vi "GetSensorInfo.vi"(11 "Sensor Serials IN":string[](array[string])) -> (0 "OK":bool, 1 "Sensor Types":string[](array[string]), 2 "Sensor DB IDs":string[](array[string]), 3 "Sensor Serials OUT":string[](array[string]), 4 "No. of Sensors":i32)   [LabVIEW 2019]
uses:
  <vilib>/Utility/file.llb/Read Delimited Spreadsheet (string).vi
panel:
  out "No Error?":bool=TRUE
  out "Numeric":i32
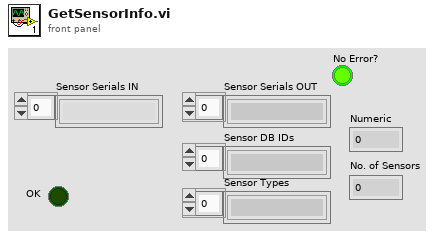
[diagram p1: front panel]
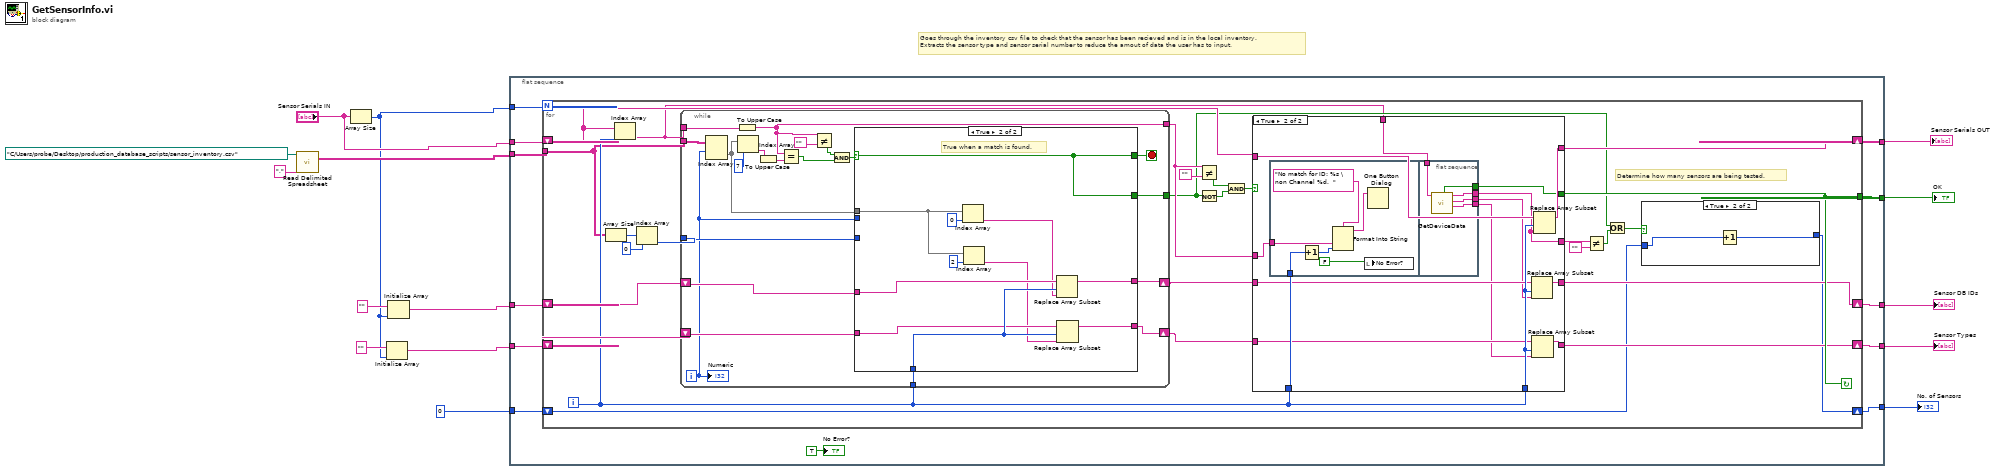
[diagram p0: block diagram]
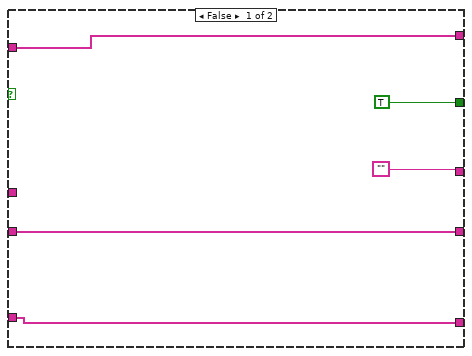
[diagram p3: hidden frame]
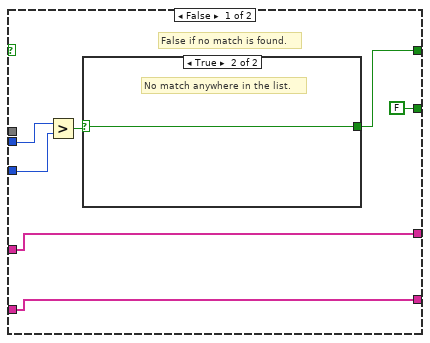
[diagram p4: hidden frame]
diagram:
  # "Goes through the inventory csv file to check that the sensor has been recieved and is in the local inventory.\nExtracts the sensor type and sensor serial number to reduce the amout of data the user has to input."
  n1 = call-poly <vilib>:"Read Delimited Spreadsheet.vi"("file path (dialog if empty)"=path "C:/Users/probe/Desktop/production_database_scripts/sensor_inventory.csv", "delimiter (\\t)"="," ("delimiter (\\t)")) -> ("all rows"=w12:string[][])  [unwired: 8 in, 5 out]
  n2 = Array Size(array="Sensor Serials IN") -> (size(s)=w9:i32)
  n3 = Initialize Array("", w9) -> (w7:string[])
  n4 = Initialize Array("", w9) -> (w8:string[])
  n5 = flat-sequence {
    tunnel: "Sensor Serials IN" -> [w27]
    tunnel: w12 -> [w26]
    tunnel: w9 -> [w25]
    tunnel: w8 -> [w24]
    tunnel: w7 -> [w23]
    tunnel: 0 -> [w17]
    tunnel: [w22] -> w6
    tunnel: [w21] -> w5
    tunnel: [w20] -> w4
    tunnel: [w19] -> w3
    tunnel: [w16] -> w1
    frame #0 {
      n6 = for {
        N: w25 -> [_]
        tunnel: w26 -> [w41]
        shift-right: [w37] -> w22
        shift-left: w24 -> [w54]
        shift-right: [w36] -> w21
        shift-left: w23 -> [w53]
        shift-right: [w47] -> w20
        shift-left: w27 -> [w48]
        tunnel: [w43] -> w19
        shift-right: [w33] -> w16
        shift-left: w17 -> [w32]
        i -> [w42]
        stop <- w43 continue-if-true
        # "Determine how many sensors are being tested."
        n7 = Array Size(array=w41) -> (size(s)=w46:i32[])
        n8 = Index Array(array=w48, index=w42) -> (element=w28:string)
        n9 = Index Array(array=w46, index=0) -> (element=w44:i32)
        n10 = while {
          tunnel: w28 -> [w107]
          tunnel: w42 -> [w103]
          tunnel: [w88] -> w40
          tunnel: [w101] -> w29
          tunnel: w44 -> [w100]
          shift-right: [w99] -> w39
          shift-left: w54 -> [w106]
          shift-right: [w102] -> w38
          shift-left: w53 -> [w105]
          tunnel: w41 -> [w97]
          i -> [w96]
          stop <- w104 stop-if-true
          n11 = Index Array(array=w97, index (row)=w96) -> (element=w95:string[])  [unwired: 1 in]
          n12 = To Upper Case(1:w107) -> (0:w88:string)
          n13 = Index Array(array=w95, index=7) -> (element=w93:string)
          n14 = To Upper Case(1:w93) -> (0:w98:string)
          n15 = Equal?(x=w88, y=w98) -> (x = y?=w90:bool)
          n16 = Not Equal?(x=w88, y="") -> (x != y?=w89:bool)
          n17 = And(x=w89, y=w90) -> (x .and. y?=w91:bool)
          n18 = case shown="True" w91 {
            selector: w91 -> [_ w117]
            tunnel: w106 -> [w114 w126]
            tunnel: w105 -> [w113 w125]
            tunnel: [w109 w117] -> w104
            tunnel: w103 -> [_ w127]
            tunnel: w95 -> [_ w124]
            tunnel: [w114 w120] -> w99
            tunnel: [w113 w119] -> w102
            tunnel: [FALSE w117] -> w101
            tunnel: w96 -> [w111 _]
            tunnel: w100 -> [w110 _]
            frame False {
              # "False if no match is found."
              n19 = Greater?(x=w111, y=w110) -> (0:w112:bool)
              n20 = case shown="True" w112 {
                selector: w112 -> [w115 w116]
                tunnel: [w115 w116] -> w109
                frame False {
                }
                frame True {
                  # "No match anywhere in the list."
                }
              }
            }
            frame True {
              # "True when a match is found."
              n21 = Index Array(array=w124, index=0) -> (element=w118:string)
              n22 = Index Array(array=w124, index=2) -> (element=w121:string)
              n23 = Replace Array Subset(array=w126, new element=w118, index=w127) -> (w120:string[])
              n24 = Replace Array Subset(array=w125, new element=w121, index=w127) -> (w119:string[])
            }
          }
          "Numeric" <- w96
        }
        n25 = Not Equal?(x=w40, y="") -> (x != y?=w50:bool)
        n26 = Not(x=w29) -> (.not. x?=w49:bool)
        n27 = And(x=w50, y=w49) -> (x .and. y?=w52:bool)
        n28 = case shown="True" w52 {
          tunnel: w42 -> [_ w73]
          tunnel: w48 -> [w62 w76]
          tunnel: [w62 w75] -> w47
          tunnel: [TRUE ("OK") w64] -> w43
          tunnel: w42 -> [_ w74]
          tunnel: w40 -> [_ w68]
          tunnel: w39 -> [w60 w72]
          tunnel: w38 -> [w59 w71]
          tunnel: [w60 w70] -> w37
          tunnel: [w59 w69] -> w36
          tunnel: ["" w65] -> w34
          tunnel: w28 -> [_ w63]
          frame False {
          }
          frame True {
            n29 = flat-sequence {
              tunnel: w74 -> [w79]
              tunnel: w68 -> [w77]
              tunnel: [w87] -> w67
              tunnel: [w86] -> w66
              tunnel: [w85] -> w65
              tunnel: [w84] -> w64
              tunnel: w63 -> [w83]
              frame #0 {
                n30 = Increment(x=w79) -> (x+1=w78:i32)
                n31 = Format Into String(format string="No match for ID: %s \non Channel %d.  " ("initial string"), w77, w78) -> (resulting string=w80:string)  [unwired: 2 in, 1 out]
                n32 = local write "No Error?"(FALSE ("Done?")) -> ()
                n33 = One Button Dialog(message=w80) -> ()  [unwired: 1 in, 1 out]
              }
              frame #1 {
                n34 = call "GetDeviceData.vi"("ID"=w83) -> ("Type 2"=w87:string, "DB Serial Number 2"=w86:string, "ID 2"=w85:string, 5:w84:bool)  [unwired: 7 in]
              }
            }
            n35 = Replace Array Subset(array=w72, new element=w66, index=w73) -> (w70:string[])
            n36 = Replace Array Subset(array=w71, new element=w67, index=w73) -> (w69:string[])
            n37 = Replace Array Subset(array=w76, new element=w65, index=w73) -> (w75:string[])
          }
        }
        n38 = Not Equal?(x=w34, y="") -> (x != y?=w30:bool)
        n39 = Or(x=w29, y=w30) -> (x .or. y?=w31:bool)
        n40 = case shown="True" w31 {
          tunnel: [w55 w57] -> w33
          tunnel: w32 -> [w55 w56]
          frame False {
          }
          frame True {
            n41 = Increment(x=w56) -> (x+1=w57:i32)
          }
        }
      }
      "No Error?" <- TRUE ("Done?")
    }
  }
  "Sensor Serials OUT" <- w4
  "Sensor DB IDs" <- w6
  "Sensor Types" <- w5
  "OK" <- w3
  "No. of Sensors" <- w1
